vi "save_zip.vi"(0 "error IO":errorcluster, 1 "Array 2":T2(array[cluster])) -> (2 "error IO 2":errorcluster, 3 "Array":path[](array[path]), 4 "Cluster":T1)   [LabVIEW 2010]
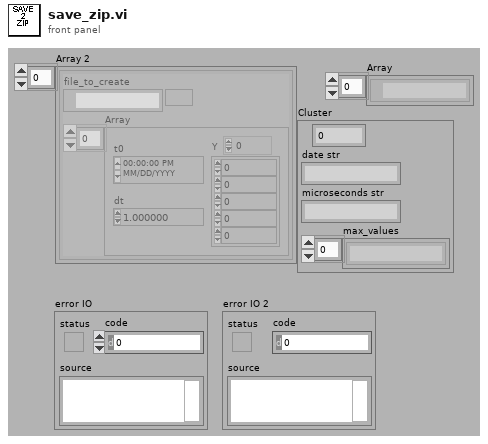
[diagram p1: front panel]
types:
  T1 = cluster{i32, "date str":string, "microseconds str":string, "max_values":string[]}
  T2 = cluster{"file_to_create":path, "Array":waveform(i16)[]}[]
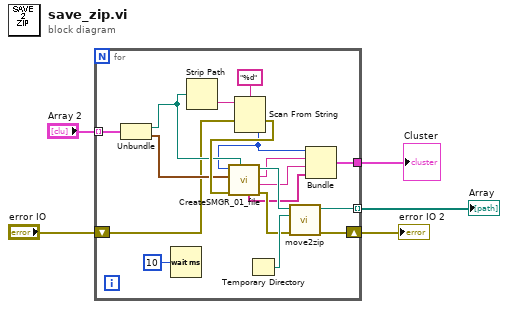
[diagram p0: block diagram]
diagram:
  n1 = for {
    tunnel: "Array 2" -> [w17] mode=indexing
    tunnel: [w13] -> w2 mode=indexing
    shift-right: [w12] -> w3
    shift-left: "error IO" -> [w14]
    tunnel: [w8] -> w4
    n2 = Unbundle(w17) -> ("file_to_create"=w16:path, "Array"=w15:waveform(i16)[])
    n3 = Wait (ms)(milliseconds to wait=u32 10) -> ()  [unwired: 1 out]
    n4 = Strip Path(path=w16) -> (name=w19:string)  [unwired: 1 out]
    n5 = Scan From String(format string="%d", input string=w19, error in=w14) -> (error out=w18:errorcluster, output 1=w7:i32)  [unwired: 2 in, 2 out]
    n6 = call "CreateSMGR_01_file.vi"("file path to write"=w16, "error in"=w18, "Waveform Graph"=w15, "meas_point"=w7) -> ("error out"=w21:errorcluster, "microseconds str"=w10:string, "date str"=w11:string, "file path out"=w22:path, "max_values"=w9:string[])  [unwired: 3 in]
    n7 = Temporary Directory() -> (w23:path)
    n8 = call "move2zip.vi"("error in"=w21, "dest dir"=w23, "source path"=w22) -> ("error out"=w12:errorcluster, "zipped path"=w13:path)  [unwired: 3 in]
    n9 = Bundle(w7, "date str"=w11, "microseconds str"=w10, "max_values"=w9) -> (w8:T1)  [unwired: 1 in]
  }
  "error IO 2" <- w3
  "Array" <- w2
  "Cluster" <- w4
